vi "Check Tags.vi"(8 "error in (no error)":errorcluster, 11 "Tags":string[](array[string])) -> (0 "error out":errorcluster, 3 "active":bool)   [LabVIEW 2020, in "Feed.lvclass"]
uses:
  <vilib>/NI_RSS/Feed/Feed.lvclass
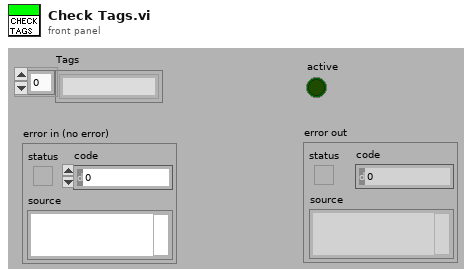
[diagram p1: front panel]
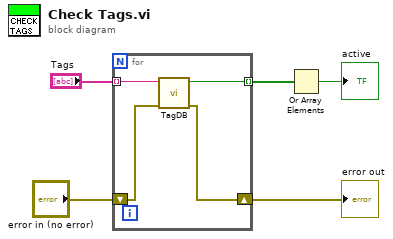
[diagram p0: block diagram]
diagram:
  n1 = for {
    tunnel: "Tags" -> [w9] mode=indexing
    shift-right: [w7] -> w3
    shift-left: "error in (no error)" -> [w8]
    tunnel: [w6] -> w2 mode=indexing
    n2 = call <vilib>:"TagDB.vi"("error in (no error)"=w8, "Tag"=w9) -> ("error out"=w7:errorcluster, "active"=w6:bool)  [unwired: 8 out]
  }
  "error out" <- w3
  n3 = Or Array Elements(Boolean array=w2) -> (logical OR=→"active":bool)
